vi "AC_Dummy_bak.vi"(3 "UR":string, 7 "Top":string, 8 "Error In":errorcluster, 10 "ML":dbl, 11 "UL":string) -> (0 "Error Out":errorcluster)   [LabVIEW 2011]
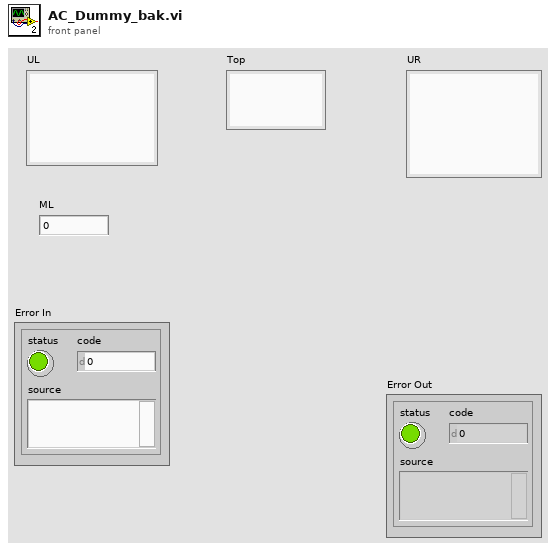
[diagram p1: front panel]
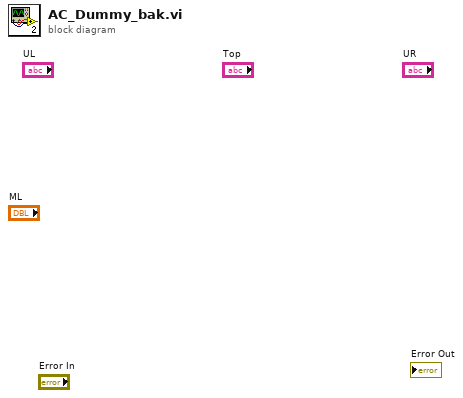
[diagram p0: block diagram]
diagram:
